vi "DestroyProtectedEvents.vi"(8 "error in (no error)":errorcluster, 11 "LMT":refnum<class "LMT.lvclass">) -> (0 "error out":errorcluster, 3 "LMT out":refnum<class "LMT.lvclass">)   [LabVIEW 2017, in "LMT.lvclass"]
doc: "JKI State Machine Objects (SMO) 1.0.0.5\nJKI - JKI\nCopyright (c) 2016, JKI"
uses:
  LMT.lvclass
  <vilib>/JKI/JKI SMO/SMO/SMO.lvclass
panel:
  # "For instructions on how to use the JKI State Machine Objects, examples and video tutorials, visit:\nhttp://jki.net/state-machine-objects/\n\nJKI State Machine Objects™\nhttp://jki.net/state-machine-objects/\nCopyright (C) 2005-2015, JKI <info@jki.net>\nALL RIGHTS RESERVED"
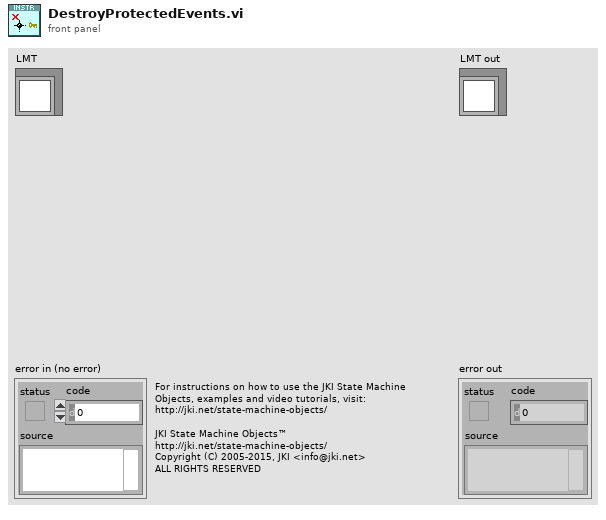
[diagram p1: front panel]
types:
  T1 = typedef "LMT.lvclass/ProtectedEvents--Cluster.ctl" = cluster{"API_Template":refnum<user-event>}
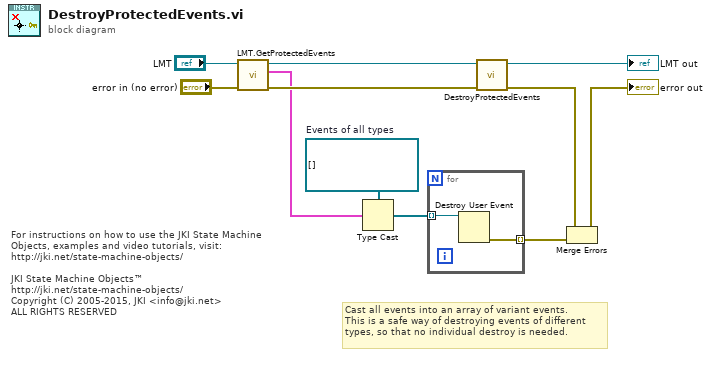
[diagram p0: block diagram]
diagram:
  w3 = refnum<user-event>[] []  # Events of all types
  # "For instructions on how to use the JKI State Machine Objects, examples and video tutorials, visit:\nhttp://jki.net/state-machine-objects/\n\nJKI State Machine Objects™\nhttp://jki.net/state-machine-objects/\nCopyright (C) 2005-2015, JKI <info@jki.net>\nALL RIGHTS RESERVED"
  # "Cast all events into an array of variant events.\nThis is a safe way of destroying events of different\ntypes, so that no individual destroy is needed."
  n1 = call "LMT.GetProtectedEvents.vi"("error in (no error)"="error in (no error)", "LMT"="LMT") -> ("error out"=w5:errorcluster, "Protected Events"=w4:T1, "LMT out"=w7:refnum<class "LMT.lvclass">)  [unwired: 7 in]
  n2 = Type Cast(type=w3, x=w4) -> (*(type *) &x=w2:refnum<user-event>[])
  n3 = for {
    tunnel: w2 -> [w13] mode=indexing
    tunnel: [w12] -> w1 mode=indexing
    n4 = Destroy User Event(user event=w13) -> (error out=w12:errorcluster)  [unwired: 1 in]
  }
  n5 = call-parent "DestroyProtectedEvents.vi"("error in (no error)"=w5, "SMO"=w7) -> ("error out"=w10:errorcluster, "SMO out"=→"LMT out":refnum<class "LMT.lvclass">)  [unwired: 8 in]
  n6 = Merge Errors(w10, w1) -> (→"error out":errorcluster)
